vi "pf_Get_Camera_Property_Bool.vi"(8 "error in (no error)":errorcluster, 10 "Property Name":string, 11 "IMAQ Session in":refnum<k11>) -> (0 "error out":errorcluster, 1 "Property Value":bool, 2 "Property Name out":string, 3 "IMAQ Session out":refnum<k11>)   [LabVIEW 2025, in "Photonfocus_Toolkit.lvlib"]
doc: "Gets the value of a Boolean type property."
uses:
  Photonfocus_Toolkit.lvlib
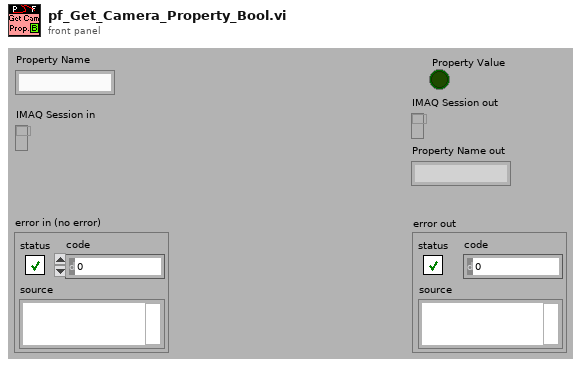
[diagram p1: front panel]
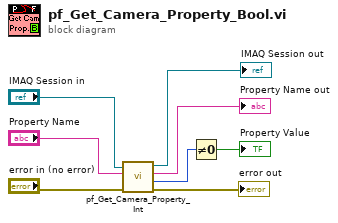
[diagram p0: block diagram]
diagram:
  n1 = call "pf_Get_Camera_Property_Int.vi"("error in (no error)"="error in (no error)", "Property Name"="Property Name", "IMAQ Session in"="IMAQ Session in") -> ("error out"=→"error out":errorcluster, "Property Value"=w2:i32, "Property Name out"=→"Property Name out":string, "IMAQ Session out"=→"IMAQ Session out":refnum<k11>)  [unwired: 5 out]
  n2 = Not Equal To 0?(x=w2) -> (x != 0?=→"Property Value":bool)
